vi "Configure Frequency.vi"   [LabVIEW 2022 SP3, in "Agilent N934X Series.lvlib"]
doc: "This is a poly VI for configure frequency VIs."
uses:
  <instrlib>/Agilent N934X Series/Agilent N934X Series.lvlib
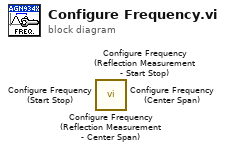
[diagram p0: block diagram]
diagram:
  n1 = call <instrlib>:"Configure Frequency (Reflection Measurement - Center Span).vi"() -> ()  [unwired: 14 in, 2 out]
  n2 = call <instrlib>:"Configure Frequency (Reflection Measurement - Start Stop).vi"() -> ()  [unwired: 14 in, 2 out]
  n3 = call <instrlib>:"Configure Frequency (Start Stop).vi"() -> ()  [unwired: 14 in, 2 out]
  n4 = call <instrlib>:"Configure Frequency (Center Span).vi"() -> ()  [unwired: 14 in, 2 out]
